vi "AlliGator Python Plugin Target Information.vi"(8 "error in (no error)":errorcluster, 11 "Script Header":string) -> (0 "error out":errorcluster, 1 "Parent Menu Locations":string[](array[string]), 2 "Function Target Types":T2[](array[typedef]), 3 "Function Target Windows":string[](array[string]))   [LabVIEW 2021, in "AlliGator Python Plugins.lvlib"]
doc: "Extracts information on the python plugin target(s)."
uses:
  AlliGator Python Plugins.lvlib
  AlliGator Python Plugin Target Type.ctl
  AlliGator Windows List.ctl
  ac9583af-a777-400e-974f-fc8935ef7273.vi
  AlliGator GUI.lvlib
panel:
  in  "Source":string
  in  "AlliGator Windows":T1
  # "see the AlliGator License on the block diagram (Ctrl+E or Window:Show Block Diagram)"
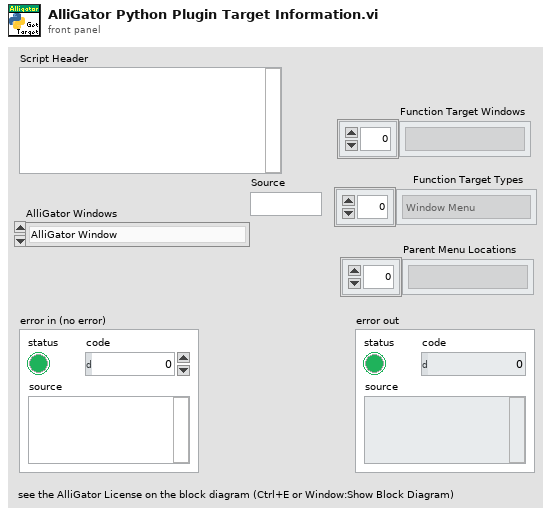
[diagram p1: front panel]
types:
  T1 = typedef "AlliGator GUI.lvlib/AlliGator Windows List.ctl" = enum16{"AlliGator Window", "Settings Window", "Notebook Window", "Dataset Information Window", "Source Image ROI Manager Window", "Phasor Plot ROI Manager Window", "Phasor Harmonic Manager Window", "Histogram Window", "Image Profile Window", "Local Decay Window", "About Window", "Batch Conversion Window", "Shot Noise Influence on Average Lifetime", "Fit Method Benchmark", "AlliGator Alias Definition"}
  T2 = typedef "AlliGator Python Plugins.lvlib/AlliGator Python Plugin Target Type.ctl" = enum16{"Undefined", "Window Menu", "Object Menu"}
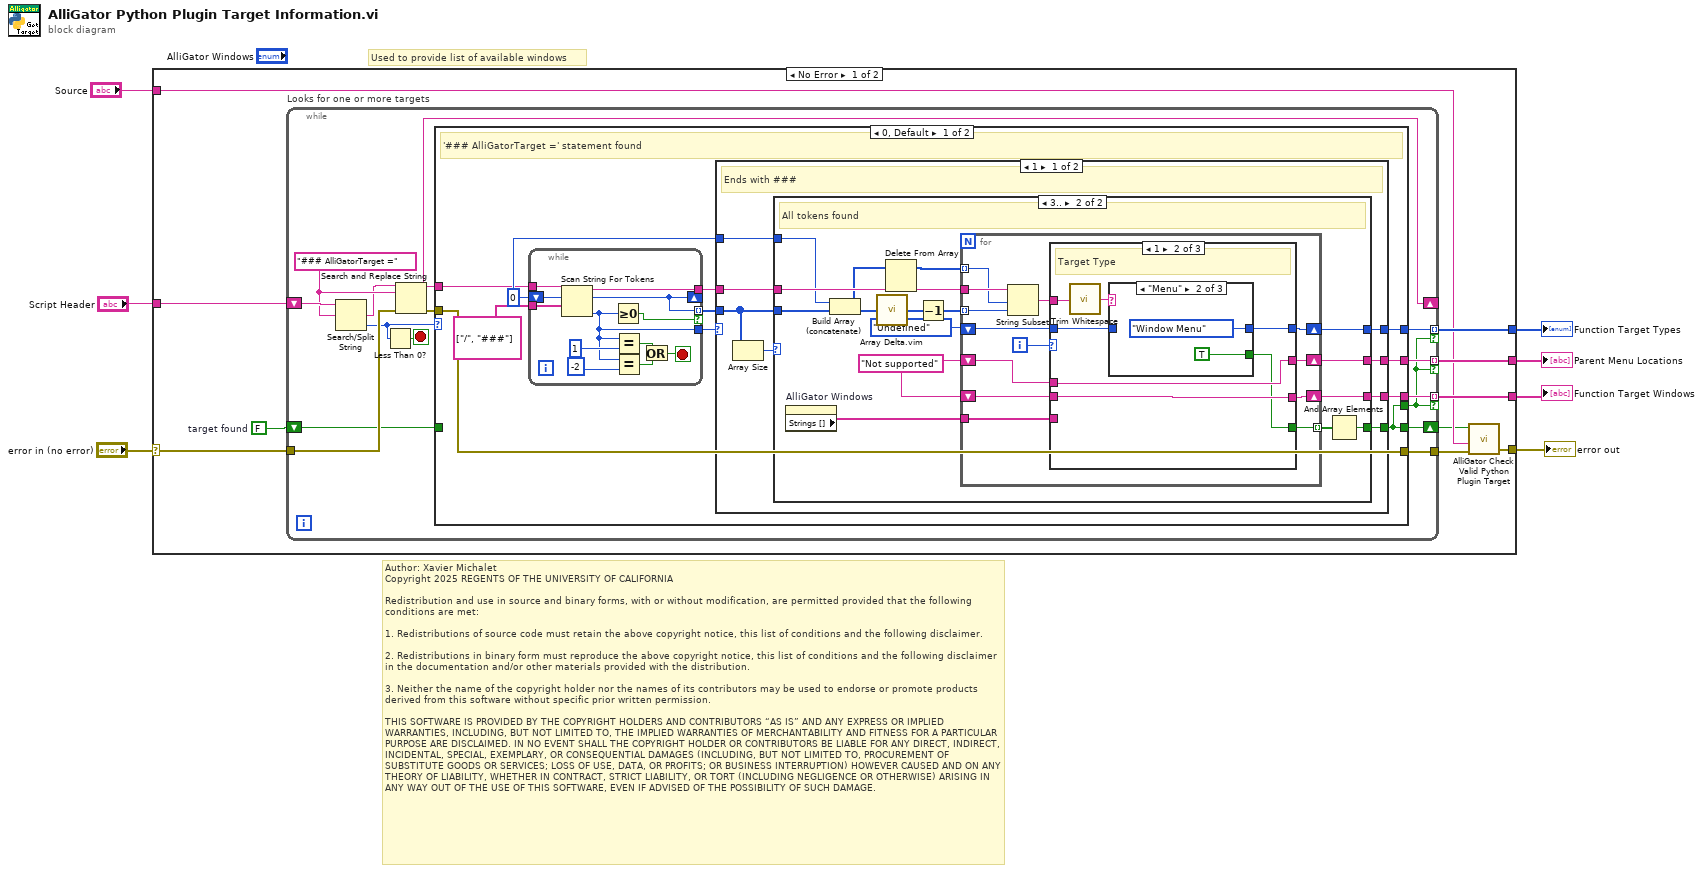
[diagram p0: block diagram]
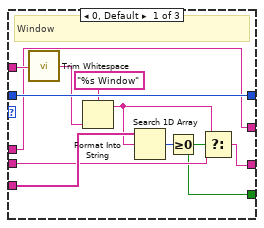
[diagram p3: hidden frame]
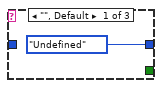
[diagram p4: hidden frame]
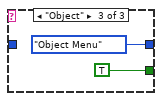
[diagram p5: hidden frame]
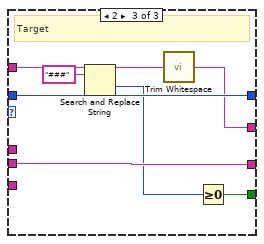
[diagram p6: hidden frame]
diagram:
  # "Author: Xavier Michalet\nCopyright 2025 REGENTS OF THE UNIVERSITY OF CALIFORNIA\n\nRedistribution and use in source and binary forms, with or without modification, are permitted provided that the following conditions are met:\n\n1. Redistributions of source code must retain the above copyright notice, this list of conditions and the following disclaimer.\n\n2. Redistributions in binary form must reproduce the above copyright notice, this list of conditions and the following disclaimer in the documentation and/or other materials provided with the distribution.\n\n3. Neither the name of the copyright holder nor the names of its contributors may be used to endorse or promote products derived from this software without specific prior written permission.\n\nTHIS SOFTWARE IS PROVIDED BY THE COPYRIGHT HOLDERS AND CONTRIBUTORS “AS IS” AND ANY EXPRESS OR IMPLIED WARRANTIES, INCLUDING, BUT NOT LIMITED TO, THE IMPLIED WARRANTIES OF MERCHANTABILITY AND FITNESS FOR A PARTICULAR PURPOSE ARE DISCLAIMED. IN NO EVENT SHALL THE COPYRIGHT HOLDER OR CONTRIBUTORS BE LIABLE FOR ANY DIRECT, INDIRECT, INCIDENTAL, SPECIAL, EXEMPLARY, OR CONSEQUENTIAL DAMAGES (INCLUDING, BUT NOT LIMITED TO, PROCUREMENT OF SUBSTITUTE GOODS OR SERVICES; LOSS OF USE, DATA, OR PROFITS; OR BUSINESS INTERRUPTION) HOWEVER CAUSED AND ON ANY THEORY OF LIABILITY, WHETHER IN CONTRACT, STRICT LIABILITY, OR TORT (INCLUDING NEGLIGENCE OR OTHERWISE) ARISING IN ANY WAY OUT OF THE USE OF THIS SOFTWARE, EVEN IF ADVISED OF THE POSSIBILITY OF SUCH DAMAGE."
  # "Used to provide list of available windows"
  n1 = case shown="No Error" "error in (no error)" {
    selector: "error in (no error)" -> [w10 w125]
    tunnel: "Script Header" -> [w14 _]
    tunnel: [w17 _] -> w5
    tunnel: [w16 _] -> w4
    tunnel: [w15 _] -> w3
    tunnel: [w12 w125] -> w1
    tunnel: "Source" -> [w13 _]
    frame No Error {
      w8 = FALSE  # target found
      n2 = while "Looks for one or more targets" {
        tunnel: [w32] -> w17 mode=indexing if=w18
        tunnel: [w31] -> w16 mode=indexing if=w18
        tunnel: w10 -> [w26]
        tunnel: [w30] -> w15 mode=indexing if=w18
        shift-right: [w20] -> _
        shift-left: w14 -> [w29]
        tunnel: [w25] -> w9
        shift-right: [w19] -> w11
        shift-left: w8 -> [w21]
        stop <- w23 stop-if-true
        w28 = "### AlliGatorTarget =" ("operators (none)")
        n3 = Search/Split String(string=w29, search string/char (-)=w28) -> (match + rest of string=w27:string, offset of match=w22:i32)  [unwired: 1 in, 1 out]
        n4 = Less Than 0?(x=w22) -> (x < 0?=w23:bool)
        n5 = Search and Replace String(input string=w27, search string=w28, error in=w26) -> (result string=w20:string, error out=w24:errorcluster)  [unwired: 5 in, 2 out]
        n6 = case shown="0, Default" w22 {
          tunnel: [w39 _] -> w32
          tunnel: [w38 _] -> w31
          tunnel: [w37 _] -> w30
          tunnel: w20 -> [w35 _]
          tunnel: [w33 w123] -> w19
          tunnel: [w34 w124] -> w25
          tunnel: w24 -> [w34 w124]
          tunnel: w21 -> [_ w123]
          tunnel: [w33 _] -> w18
          frame 0, Default {
            w36 = 0 ("offset past token")
            # "'### AlliGatorTarget =' statement found"
            n7 = while {
              tunnel: w35 -> [w122]
              tunnel: string[] ["/", "###"] ("operators (none)") -> [w120]
              tunnel: [w112] -> w42 mode=indexing if=w111
              tunnel: [w114] -> w41
              tunnel: [w113] -> w40
              shift-right: [w112] -> _
              shift-left: w36 -> [w121]
              stop <- w117 stop-if-true
              n8 = Scan String For Tokens(7:w120, 8:w121, 9:w122) -> (0:w114:i32, 2:w112:i32, 3:w113:string)  [unwired: 3 in, 1 out]
              n9 = Greater Or Equal To 0?(x=w114) -> (x >= 0?=w111:bool)
              n10 = Equal?(x=w114, y=1) -> (x = y?=w115:bool)
              n11 = Equal?(x=w114, y=-2) -> (x = y?=w118:bool)
              n12 = Or(x=w115, y=w118) -> (x .or. y?=w117:bool)
            }
            n13 = case shown="1" w41 {
              tunnel: w42 -> [w50 _]
              tunnel: w40 -> [w49 _]
              tunnel: w36 -> [w48 _]
              tunnel: [w47 _] -> w39
              tunnel: [w46 _] -> w38
              tunnel: [w45 _] -> w37
              tunnel: [w44 _] -> w33
              frame 1 {
                # "Ends with ###"
                n14 = Array Size(array=w50) -> (size(s)=w51:i32)
                n15 = case shown="3.." w51 {
                  tunnel: w50 -> [_ w60]
                  tunnel: w49 -> [_ w66]
                  tunnel: w48 -> [_ w59]
                  tunnel: [_ w64] -> w47
                  tunnel: [_ w61] -> w46
                  tunnel: [_ w56] -> w45
                  tunnel: [_ w52] -> w44
                  frame 0, Default {
                    # "Missing '/'"
                  }
                  frame 3.. {
                    w55 = "Not supported"
                    # "All tokens found"
                    n16 = property on="AlliGator Windows" class="Enum (strict)"() -> ("Strings []"=w63:string[])  [unwired: 2 in, 2 out]
                    n17 = Build Array (concatenate)(w59, w60) -> (w58:i32[])
                    n18 = call "Array Delta.vim"("A"=w58) -> ("A[i+1]-A[i]"=w65:i32[])  [unwired: 8 in]
                    n19 = Delete From Array(array=w58) -> (array with subset deleted=w57:i32[])  [unwired: 2 in, 1 out]
                    n20 = Decrement(x=w65) -> (x-1=w54:i32[])
                    n21 = for {
                      tunnel: w66 -> [w79]
                      tunnel: w54 -> [w78] mode=indexing
                      shift-right: [w75] -> w64
                      shift-left: AlliGator_Python_Plugin_Target_Type."Undefined" ("Function Target Type") -> [w74]
                      tunnel: w63 -> [w73]
                      shift-right: [w72] -> w61
                      shift-left: w55 -> [w71]
                      tunnel: w57 -> [w70] mode=indexing
                      shift-right: [w69] -> w56
                      shift-left: w55 -> [w68]
                      tunnel: [w67] -> w53 mode=indexing
                      i -> [w77]
                      n22 = String Subset(string=w79, offset (0)=w70, length (rest)=w78) -> (substring=w76:string)
                      n23 = case shown="1" w77 {
                        tunnel: w76 -> [w90 w97 w107]
                        tunnel: [w89 w95 w109] -> w75
                        tunnel: w74 -> [w89 w94 w109]
                        tunnel: w73 -> [w86 _ _]
                        tunnel: [w83 w93 w110] -> w72
                        tunnel: w71 -> [w82 w93 w110]
                        tunnel: [w81 w92 w108] -> w69
                        tunnel: w68 -> [w81 w92 _]
                        tunnel: [w80 w91 w103] -> w67
                        frame 0, Default {
                          # "Window"
                          n24 = call <vilib>:"Trim Whitespace.vi"("string"=w90) -> ("trimmed string"=w87:string)  [unwired: 1 in]
                          n25 = Format Into String(format string="%s Window", w87) -> (resulting string=w84:string)  [unwired: 2 in, 1 out]
                          n26 = Search 1D Array(1D array=w86, element=w84) -> (index of element=w85:i32)  [unwired: 1 in]
                          n27 = Greater Or Equal To 0?(x=w85) -> (x >= 0?=w80:bool)
                          n28 = Select(t=w84, s=w80, f=w82) -> (s? t:f=w83:string)
                        }
                        frame 1 {
                          # "Target Type"
                          n29 = call <vilib>:"Trim Whitespace.vi"("string"=w97) -> ("trimmed string"=w96:string)  [unwired: 1 in]
                          n30 = case shown="\"Menu\"" w96 {
                            tunnel: [AlliGator_Python_Plugin_Target_Type."Undefined" ("Function Target Type") AlliGator_Python_Plugin_Target_Type."Window Menu" ("Function Target Type") AlliGator_Python_Plugin_Target_Type."Object Menu" ("Function Target Type")] -> w95
                            tunnel: w94 -> [_ _ _]
                            tunnel: [_ TRUE TRUE] -> w91
                            frame "", Default {
                            }
                            frame "Menu" {
                            }
                            frame "Object" {
                            }
                          }
                        }
                        frame 2 {
                          # "Target"
                          n31 = Search and Replace String(input string=w107, search string="###") -> (result string=w105:string, offset past replacement=w104:i32)  [unwired: 6 in, 2 out]
                          n32 = call <vilib>:"Trim Whitespace.vi"("string"=w105) -> ("trimmed string"=w108:string)  [unwired: 1 in]
                          n33 = Greater Or Equal To 0?(x=w104) -> (x >= 0?=w103:bool)
                        }
                      }
                    }
                    n34 = And Array Elements(Boolean array=w53) -> (logical AND=w52:bool)
                  }
                }
              }
              frame -2, Default {
                # "Missing End of AlliGatorTarget Statement '###'"
              }
            }
          }
          frame -1 {
            # "Missing '### AlliGatorTarget =' Statement"
          }
        }
      }
      n35 = call "AlliGator Check Valid Python Plugin Target.vi"("error in (no error)"=w9, "Source"=w13, "Target Found?"=w11) -> ("error out"=w12:errorcluster)  [unwired: 8 in]
    }
    frame Error {
    }
  }
  "error out" <- w1
  "Function Target Windows" <- w4
  "Function Target Types" <- w5
  "Parent Menu Locations" <- w3
